vi "Test UDP launcher.vi"() -> ()   [LabVIEW 2021]
uses:
  <vilib>/Utility/LVLibp/NI_PackedLibraryUtility.lvlib
panel:
  out "data out":string
  in  "stop":bool
  out "error out 3":errorcluster={"status"=TRUE, "code"=56, "source"="UDP Read in Test UDP launcher.vi"}
  out "error out 2":errorcluster
  out "qualified names":string[](array[string])=["CIFTemplatePlugin.lvlibp:Energize.vi", "CIFTemplatePlugin.lvlibp:Launch.vi"]
  in  "Linux":path=path "/home/lvuser/natinst/bin/CIFTemplatePlugin.lvlibp"
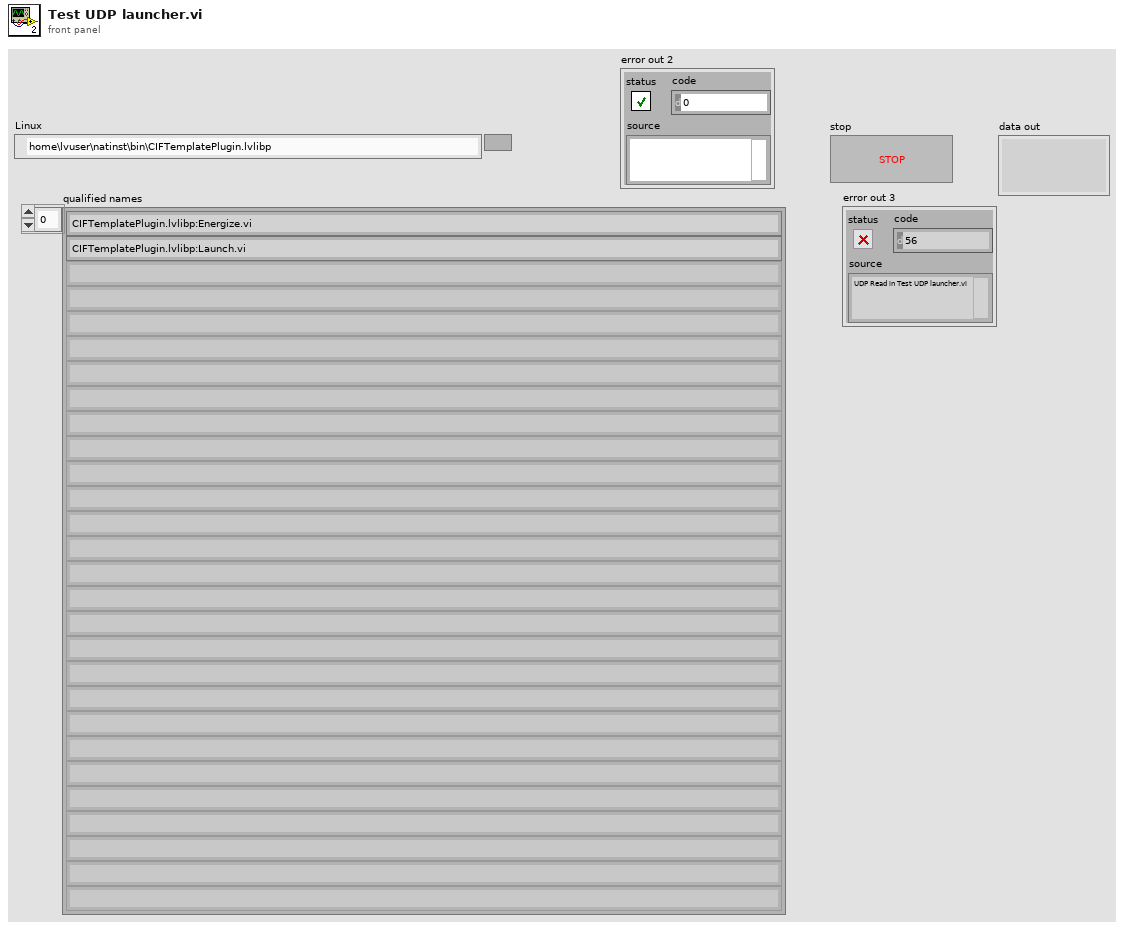
[diagram p1: front panel]
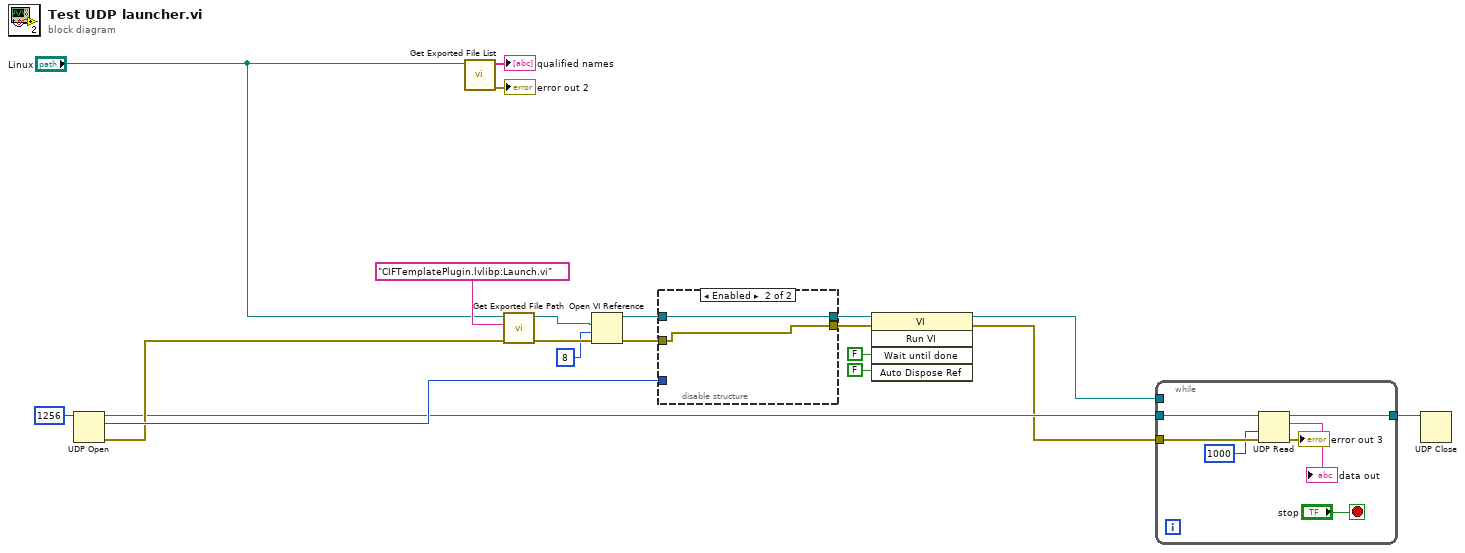
[diagram p0: block diagram]
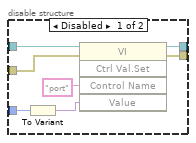
[diagram p2: hidden frame]
diagram:
  n1 = UDP Open(11:u16 1256 ("port")) -> (port=w15:refnum<k16>, 0:w16:errorcluster, 2:w17:u16)  [unwired: 4 in]
  n2 = call <vilib>:"Get Exported File List.vi"("packed library path"="Linux") -> ("error out"=→"error out 2":errorcluster, "qualified names"=→"qualified names":string[])  [unwired: 8 in, 1 out]
  n3 = call <vilib>:"Get Exported File Path.vi"("error in (no error)"=w16, "qualified name"="CIFTemplatePlugin.lvlibp:Launch.vi", "packed library path"="Linux") -> ("error out"=w10:errorcluster, "path"=w9:path)  [unwired: 7 in]
  n4 = Open VI Reference(vi path=w9, options=8, error in (no error)=w10) -> (vi reference=w3:refnum<vi>, error out=w12:errorcluster)  [unwired: 3 in]
  n5 = disable-structure shown="Enabled" {
    disable-tunnel: w17 -> [w27 _]
    disable-tunnel: [w24 w28] -> w4
    disable-tunnel: [w23 w29] -> w5
    disable-tunnel: w12 -> [w22 w28]
    disable-tunnel: w3 -> [w21 w29]
    frame Disabled {
      n6 = To Variant(anything=w27) -> (Variant=w26:variant)
      n7 = invoke class="VI" method="Ctrl Val.Set"(reference=w21, error in=w22, "Control Name"="port", "Value"=w26) -> (reference out=w23:refnum<vi>, error out=w24:errorcluster)  [unwired: 1 in, 3 out]
    }
    frame Enabled {
    }
  }
  n8 = invoke class="VI" method="Run VI"(reference=w5, error in=w4, "Wait until done"=FALSE ("Wait Until Done"), "Auto Dispose Ref"=FALSE ("Auto Dispose Reference")) -> (reference out=w1:refnum<vi>, error out=w6:errorcluster)  [unwired: 1 in, 3 out]
  n9 = while {
    tunnel: w15 -> [w36]
    tunnel: w6 -> [w35]
    tunnel: [w31] -> w8
    tunnel: w1 -> [_]
    stop <- "stop" stop-if-true
    n10 = UDP Read(connection ID=w36, timeout ms (25000)=1000, 8:w35) -> (data out=→"data out":string, error out=→"error out 3":errorcluster, 3:w31:refnum<k16>)  [unwired: 1 in, 2 out]
  }
  n11 = UDP Close(connection ID=w8) -> ()  [unwired: 1 in, 2 out]
